vi "写数值转字符协议.vi"(9 "枚举":enum16{"16位", "32位"}(ring)=enum."32位", 10 "输入数值":i32, 11 "输入地址":i32) -> (2 "返回字节数":u16, 3 "连接的字符串":string)   [LabVIEW 2018]
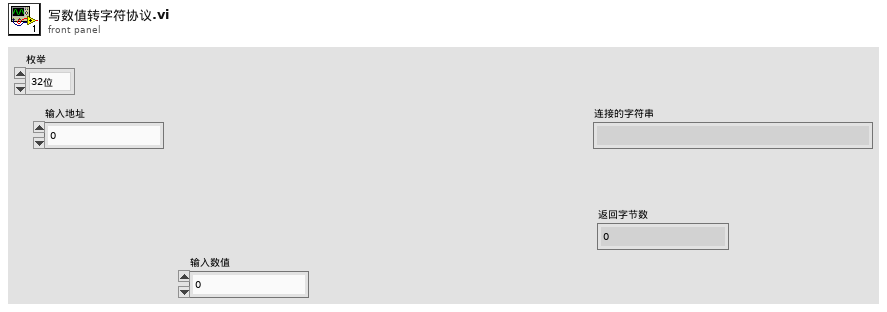
[diagram p1: front panel]
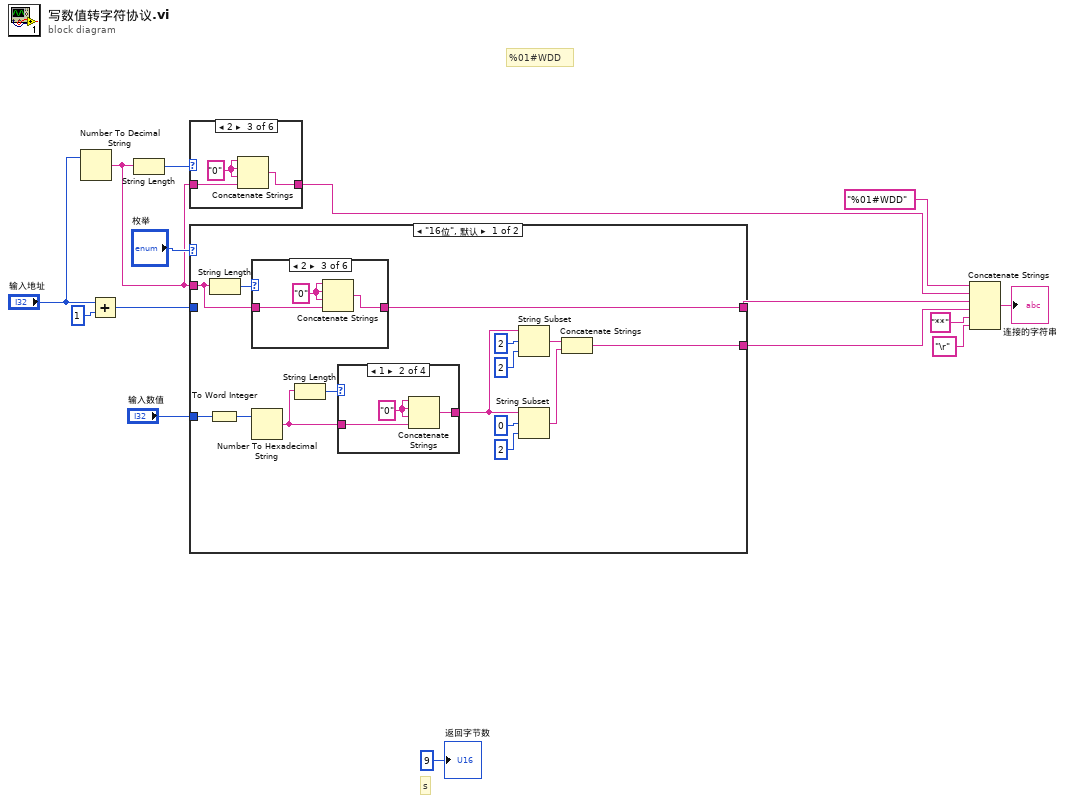
[diagram p0: block diagram]
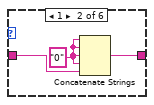
[diagram p3: hidden frame]
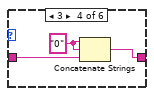
[diagram p4: hidden frame]
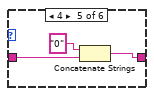
[diagram p5: hidden frame]
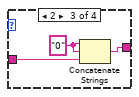
[diagram p8: hidden frame]
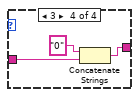
[diagram p9: hidden frame]
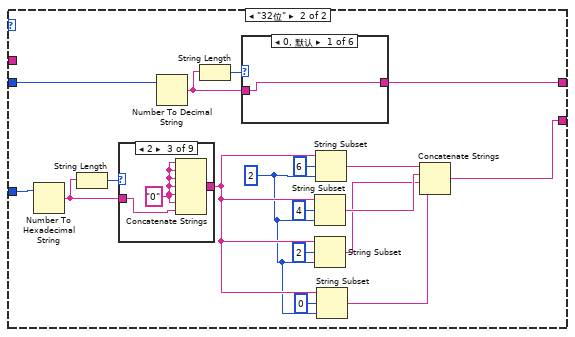
[diagram p10: hidden frame]
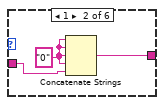
[diagram p11: hidden frame]
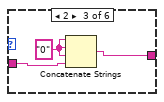
[diagram p12: hidden frame]
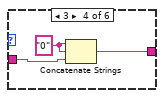
[diagram p13: hidden frame]
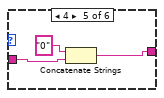
[diagram p14: hidden frame]
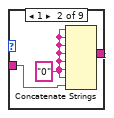
[diagram p17: hidden frame]
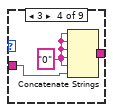
[diagram p18: hidden frame]
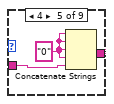
[diagram p19: hidden frame]
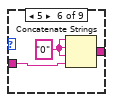
[diagram p20: hidden frame]
diagram:
  # "s"
  # "%01#WDD"
  n1 = Number To Decimal String(number="输入地址") -> (decimal integer string=w5:string)  [unwired: 1 in]
  n2 = Add(x="输入地址", y=1) -> (x+y=w1:i32)
  n3 = String Length(string=w5) -> (length=w14:i32)
  n4 = case shown="2" w14 {
    tunnel: w5 -> [w16 w19 w22 w25 w28 w29]
    tunnel: [w16 w17 w20 w23 w26 w29] -> w13
    frame 0, Default {
    }
    frame 1 {
      w18 = "0" ("字符串")
      n5 = Concatenate Strings(w18, w18, w18, w18, w19) -> (w17:string)
    }
    frame 2 {
      w21 = "0" ("字符串")
      n6 = Concatenate Strings(w21, w21, w21, w22) -> (w20:string)
    }
    frame 3 {
      w24 = "0" ("字符串")
      n7 = Concatenate Strings(w24, w24, w25) -> (w23:string)
    }
    frame 4 {
      n8 = Concatenate Strings("0" ("字符串"), w28) -> (w26:string)
    }
    frame 5 {
    }
  }
  n9 = case shown="\"16位\", 默认" "枚举" {
    tunnel: [w36 w72] -> w8
    tunnel: "输入数值" -> [w34 w85]
    tunnel: w5 -> [w31 _]
    tunnel: [w30 w79] -> w4
    tunnel: w1 -> [_ w82]
    frame "16位", Default {
      n10 = To Word Integer(number=w34) -> (16bit integer=w33:i16)
      n11 = String Length(string=w31) -> (length=w32:i32)
      n12 = case shown="2" w32 {
        tunnel: w31 -> [_ w47 w50 w53 w56 w57]
        tunnel: [_ w45 w48 w51 w54 w57] -> w30
        frame 0, Default {
        }
        frame 1 {
          w46 = "0" ("字符串")
          n13 = Concatenate Strings(w46, w46, w46, w46, w47) -> (w45:string)
        }
        frame 2 {
          w49 = "0" ("字符串")
          n14 = Concatenate Strings(w49, w49, w49, w50) -> (w48:string)
        }
        frame 3 {
          w52 = "0" ("字符串")
          n15 = Concatenate Strings(w52, w52, w53) -> (w51:string)
        }
        frame 4 {
          n16 = Concatenate Strings("0" ("字符串"), w56) -> (w54:string)
        }
        frame 5 {
        }
      }
      n17 = Number To Hexadecimal String(2:w33) -> (0:w35:string)  [unwired: 1 in]
      n18 = String Length(string=w35) -> (length=w44:i32)
      n19 = case shown="1" w44 {
        tunnel: w35 -> [w58 w61 w64 w67]
        tunnel: [w58 w59 w62 w65] -> w41
        frame 0, Default {
        }
        frame 1 {
          w60 = "0" ("字符串")
          n20 = Concatenate Strings(w60, w60, w60, w61) -> (w59:string)
        }
        frame 2 {
          w63 = "0" ("字符串")
          n21 = Concatenate Strings(w63, w63, w64) -> (w62:string)
        }
        frame 3 {
          n22 = Concatenate Strings("0" ("字符串"), w67) -> (w65:string)
        }
      }
      n23 = String Subset(string=w41, offset (0)=2 ("偏移量(0)"), length (rest)=2 ("长度（剩余）")) -> (substring=w38:string)
      n24 = String Subset(string=w41, offset (0)=0 ("偏移量(0)"), length (rest)=2 ("长度（剩余）")) -> (substring=w37:string)
      n25 = Concatenate Strings(w38, w37) -> (w36:string)
    }
    frame "32位" {
      w77 = 2 ("长度（剩余）")
      n26 = Number To Hexadecimal String(2:w85) -> (0:w83:string)  [unwired: 1 in]
      n27 = String Length(string=w83) -> (length=w84:i32)
      n28 = case shown="2" w84 {
        tunnel: w83 -> [w100 w102 w105 w109 w111 w115 w117 w120 w122]
        tunnel: [w100 w101 w106 w107 w112 w113 w116 w119 w122] -> w78
        frame 0, Default {
        }
        frame 1 {
          w103 = "0" ("字符串")
          n29 = Concatenate Strings(w103, w103, w103, w103, w103, w103, w103, w102) -> (w101:string)
        }
        frame 2 {
          w104 = "0" ("字符串")
          n30 = Concatenate Strings(w104, w104, w104, w104, w104, w104, w105) -> (w106:string)
        }
        frame 3 {
          w108 = "0" ("字符串")
          n31 = Concatenate Strings(w108, w108, w108, w108, w108, w109) -> (w107:string)
        }
        frame 4 {
          w110 = "0" ("字符串")
          n32 = Concatenate Strings(w110, w110, w110, w110, w111) -> (w112:string)
        }
        frame 5 {
          w114 = "0" ("字符串")
          n33 = Concatenate Strings(w114, w114, w114, w115) -> (w113:string)
        }
        frame 6 {
          w118 = "0" ("字符串")
          n34 = Concatenate Strings(w118, w118, w117) -> (w116:string)
        }
        frame 7 {
          n35 = Concatenate Strings("0" ("字符串"), w120) -> (w119:string)
        }
        frame 8 {
        }
      }
      n36 = Number To Decimal String(number=w82) -> (decimal integer string=w80:string)  [unwired: 1 in]
      n37 = String Length(string=w80) -> (length=w81:i32)
      n38 = case shown="0, 默认" w81 {
        tunnel: w80 -> [w86 w89 w92 w95 w98 w99]
        tunnel: [w86 w87 w90 w93 w96 w99] -> w79
        frame 0, Default {
        }
        frame 1 {
          w88 = "0" ("字符串")
          n39 = Concatenate Strings(w88, w88, w88, w88, w89) -> (w87:string)
        }
        frame 2 {
          w91 = "0" ("字符串")
          n40 = Concatenate Strings(w91, w91, w91, w92) -> (w90:string)
        }
        frame 3 {
          w94 = "0" ("字符串")
          n41 = Concatenate Strings(w94, w94, w95) -> (w93:string)
        }
        frame 4 {
          n42 = Concatenate Strings("0" ("字符串"), w98) -> (w96:string)
        }
        frame 5 {
        }
      }
      n43 = String Subset(string=w78, offset (0)=4 ("偏移量(0)"), length (rest)=w77) -> (substring=w70:string)
      n44 = String Subset(string=w78, offset (0)=2 ("偏移量(0)"), length (rest)=w77) -> (substring=w69:string)
      n45 = String Subset(string=w78, offset (0)=6 ("偏移量(0)"), length (rest)=w77) -> (substring=w71:string)
      n46 = String Subset(string=w78, offset (0)=0 ("偏移量(0)"), length (rest)=w77) -> (substring=w68:string)
      n47 = Concatenate Strings(w71, w70, w69, w68) -> (w72:string)
    }
  }
  n48 = Concatenate Strings("%01#WDD" ("字符串"), w13, w4, w8, "**" ("字符串"), "\r" ("字符串")) -> (→"连接的字符串":string)
  "返回字节数" <- u16 9 ("返回字节数")
